vi "RT_MAIN.vi"() -> ()   [LabVIEW 2019]
uses:
  <vilib>/Platform/TimedLoop/XDataNode/timing_clust.ctl
  <vilib>/Platform/TimedLoop/XDataNode/nitl_modes.ctl
  <vilib>/Platform/TimedLoop/XDataNode/wakeup.ctl
  <vilib>/FPGAPlugInAG/myRIO-1900/niLvFpga_Open_myRIO-1900.vi
  <vilib>/rvi/interface/common/dynamic/niFpgaDynamicAddResources.vi
  <vilib>/Utility/error.llb/Error Cluster From Error Code.vi
  <vilib>/rvi/errors/niLvFpgaAdjustHostInterfaceError.vi
  <vilib>/rvi/interface/common/niFpgaWaitOnOcc.vi
  <vilib>/FPGAPlugInAG/Dynamic/niLvFpga_Run_Dynamic.vi
  <vilib>/FPGAPlugInAG/Dynamic/niLvFpga_Close_Dynamic.vi
  <vilib>/platform/TimedLoop/XDataNode/XDataNode.xnode
  <vilib>/rvi/interface/nirviOpenFPGA/nirviOpenFPGA.xnode
  FPGA Bitfiles/lab4ok_FPGATarget_MAINFPGA_mzQeS8+GuA0.lvbitx
  MAIN_FPGA.vi
  <vilib>/rvi/interface/nirviReadWriteControl/nirviReadWriteControl.xnode
  <vilib>/rvi/interface/nirviMethod/nirviMethod.xnode
  <vilib>/rvi/interface/nirviCloseFPGA/nirviCloseFPGA.xnode
  <vilib>/rvi/interface/Simulation/niFpgaSimulationCallBeginRW.vi
  <vilib>/rvi/errors/niLvFpgaMergeErrorWithErrorCode.vi
  <vilib>/Platform/TimedLoop/XDataNode/XDNodeRunTimeDep.lvlib
  <vilib>/FPGAPlugInAG/Dynamic/niLvFpga_ReadFifo_Dynamic.vi
  NiFpgaLv.dll
  <vilib>/FPGAPlugInAG/Dynamic/niLvFpga_ConfigureFifo_Dynamic.vi
  <vilib>/FPGAPlugInAG/Dynamic/niLvFpga_StartFifo_Dynamic.vi
panel:
  out "LatestAccTimeout":bool
  out "Waveform Graph":i16[][](graph)
  in  "stop":bool
  out "Data Recieved":i32
  in  "TriggerLevelX":i16
  in  "TriggerLevelY":i16
  in  "TriggerLevelZ":i16
  in  "Monitoring?":bool
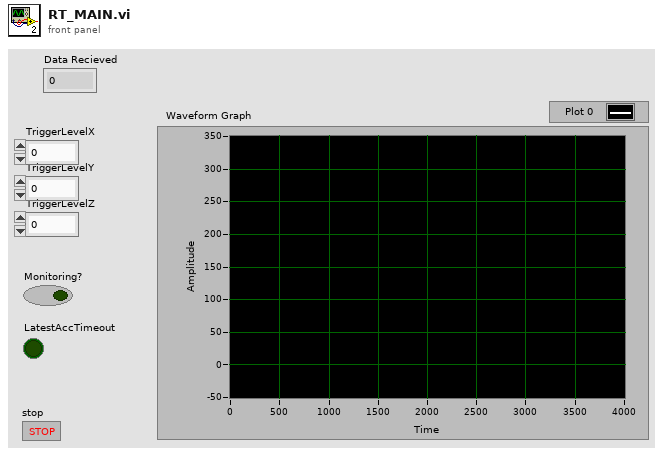
[diagram p1: front panel]
types:
  T1 = typedef "XDNodeRunTimeDep.lvlib/timing_clust.ctl" = cluster{"Expected End [f-1]":u64, "Actual End [f-1]":u64, "Finished Late? [f-1]":bool, "Expected End [i-1]":u64, "Actual End [i-1]":u64, "Finished Late? [i-1]":bool, "Expected Start [i]":u64, "Actual Start [i]":u64, "Expected Start [f]":u64, "Actual Start [f]":u64, "Source Name":string, "Structure Name":string, "Period":i64, "Deadline":i64, "Offset":i64, "Start":i64, "Priority":i32, "Timeout":i32, "Mode":T2, "Wakeup Reason":T3, "Error":errorcluster, "Source Type":string, "Secondary Source Type":string, "Global End Time":u64, "Global Start Time":u64, "Frame Duration":u64, "Iteration Duration":u64, "Assigned CPU":i32, "I/O Scan Engine Mode":u32}
  T2 = typedef "XDNodeRunTimeDep.lvlib/nitl_modes.ctl" = enum32{"No Change", "Process missed periods, maintain original phase", "Discard missed periods, maintain original phase", "Process missed periods, ignore original phase", "Discard missed periods, ignore original phase"}
  T3 = typedef "XDNodeRunTimeDep.lvlib/wakeup.ctl" = enum32{"Normal", "Aborted", "Asynchronous wakeup", "Timing source error", "Timed loop error", "Timeout"}
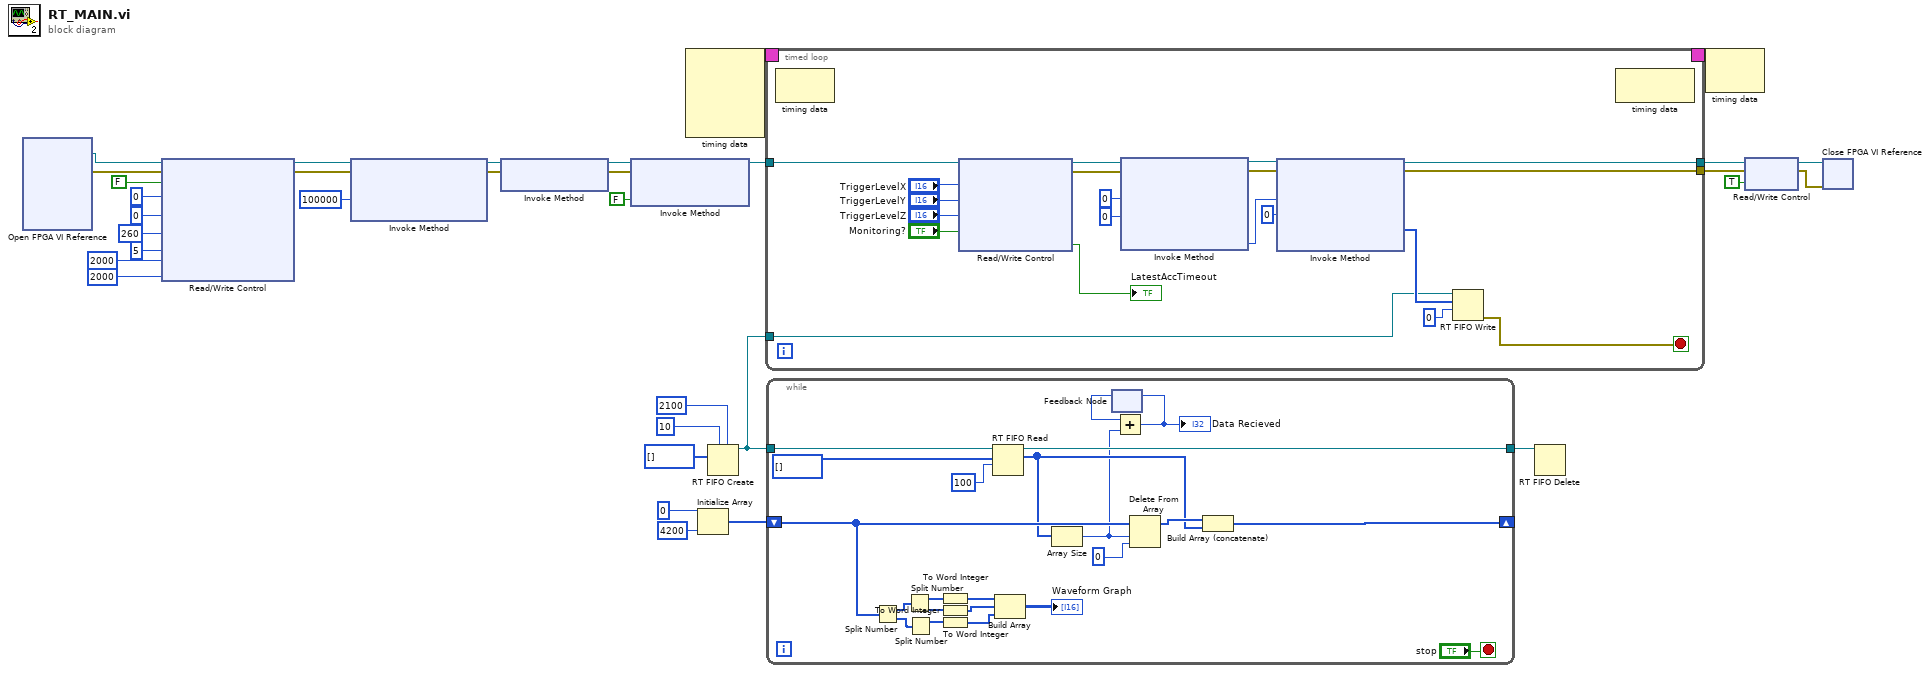
[diagram p0: block diagram]
diagram:
  n1 = xnode "Open FPGA VI Reference"() -> ("FPGA VI Reference Out"=w2:refnum<k20>, "error out"=w1:errorcluster)  [unwired: 2 in]
  n2 = xnode "Read/Write Control"("FPGA VI Reference In"=w2, "error in"=w1, "stop"=FALSE, "TriggerX"=i16 0, "TriggerY"=i16 0, "TriggerZ"=i16 260, "SamplesOverTreshold"=u8 5, "PretriggerLenght"=u16 2000, "PosttriggerLenght"=u16 2000) -> ("FPGA VI Reference Out"=w26:refnum<k20>, "error out"=w22:errorcluster)
  n3 = xnode "Invoke Method"("FPGA VI Reference In"=w26, "error in"=w22, "Requested Depth"=u32 100000) -> ("FPGA VI Reference Out"=w24:refnum<k20>, "error out"=w21:errorcluster)  [unwired: 1 out]
  n4 = xnode "Invoke Method"("FPGA VI Reference In"=w24, "error in"=w21) -> ("FPGA VI Reference Out"=w23:refnum<k20>, "error out"=w20:errorcluster)
  n5 = xnode "Invoke Method"("FPGA VI Reference In"=w23, "error in"=w20, "Wait Until Done (F)"=FALSE) -> ("FPGA VI Reference Out"=w19:refnum<k20>)  [unwired: 1 out]
  n6 = node-c288() -> (w33:T1)  [unwired: 4 in]
  n7 = Initialize Array(u64 0 ("element"), 4200 ("dimension size")) -> (w4:u64[])
  n8 = RT FIFO Create(1:u64[] [] ("Data"), 4:u32 10 ("size (10)"), 6:u32 2100 ("elements in array (1)")) -> (8:w7:refnum<k33>)  [unwired: 5 in, 2 out]
  n9 = timed-loop {
    timing: w33 -> [_]
    timing-out: [_] -> w32
    tunnel: w19 -> [w53]
    tunnel: [w52] -> w18
    tunnel: [w51] -> w14
    tunnel: w7 -> [w37]
    stop <- w35 stop-if-true
    n10 = node-c288() -> ()  [unwired: 1 in, 1 out]
    n11 = xnode "Read/Write Control"("FPGA VI Reference In"=w53, "TriggerX"="TriggerLevelX", "TriggerY"="TriggerLevelY", "TriggerZ"="TriggerLevelZ", "Monitoring?"="Monitoring?") -> ("FPGA VI Reference Out"=w47:refnum<k20>, "error out"=w45:errorcluster, "LatestAccTimeout"=→"LatestAccTimeout":bool)  [unwired: 1 in]
    n12 = xnode "Invoke Method"("FPGA VI Reference In"=w47, "error in"=w45, "Number of Elements"=u32 0, "Timeout (ms)"=0) -> ("FPGA VI Reference Out"=w46:refnum<k20>, "error out"=w44:errorcluster, "Elements Remaining"=w41:u32)  [unwired: 1 out]
    n13 = xnode "Invoke Method"("FPGA VI Reference In"=w46, "error in"=w44, "Number of Elements"=w41, "Timeout (ms)"=0) -> ("FPGA VI Reference Out"=w52:refnum<k20>, "error out"=w51:errorcluster, "Data"=w38:u64[])  [unwired: 1 out]
    n14 = RT FIFO Write(0:w37, 1:w38, 2:0 ("timeout in ms (0)")) -> (11:w35:errorcluster)  [unwired: 2 in, 3 out]
    n15 = node-c288() -> ()  [unwired: 1 in, 1 out]
  }
  n16 = while {
    tunnel: w7 -> [w77]
    tunnel: [w60] -> w8
    shift-right: [w59] -> _
    shift-left: w4 -> [w63]
    stop <- "stop" stop-if-true
    n17 = Split Number(x=w63) -> (hi(x)=w72:u32[], lo(x)=w65:u32[])
    n18 = Split Number(x=w72) -> (hi(x)=w71:u16[], lo(x)=w69:u16[])
    n19 = Split Number(x=w65) -> (hi(x)=w70:u16[])  [unwired: 1 out]
    n20 = To Word Integer(number=w71) -> (16bit integer=w68:i16[])
    n21 = To Word Integer(number=w69) -> (16bit integer=w67:i16[])
    n22 = To Word Integer(number=w70) -> (16bit integer=w66:i16[])
    n23 = RT FIFO Read(0:w77, 1:u64[] [] ("element"), 2:100 ("timeout in ms (0)")) -> (8:w60:refnum<k33>, 9:w61:u64[])  [unwired: 1 in, 3 out]
    n24 = Build Array(w68, w67, w66) -> (→"Waveform Graph":i16[][])
    n25 = Array Size(array=w61) -> (size(s)=w58:i32)
    n26 = feedback #1() -> (w56:i32)  [unwired: 1 in]
    n27 = Add(x=w56, y=w58) -> (x+y=w57:i32)
    "Data Recieved" <- w57
    n28 = feedback-in #1(w57) -> ()
    n29 = Delete From Array(array=w63, length=w58, index=0) -> (array with subset deleted=w73:u64[])  [unwired: 1 out]
    n30 = Build Array (concatenate)(w73, w61) -> (w59:u64[])
  }
  n31 = RT FIFO Delete(0:w8) -> ()  [unwired: 2 in, 1 out]
  n32 = node-c288(w32) -> ()  [unwired: 1 out]
  n33 = xnode "Read/Write Control"("FPGA VI Reference In"=w18, "error in"=w14, "stop"=TRUE) -> ("FPGA VI Reference Out"=w16:refnum<k20>, "error out"=w15:errorcluster)
  n34 = xnode "Close FPGA VI Reference"("FPGA VI Reference In"=w16, "error in"=w15) -> ()  [unwired: 1 out]
